vi "Flush if true.vi"(8 "error in":errorcluster, 10 "Bytes at port > X":bool, 11 "port in":refnum<visa-resource-name>) -> (0 "error out":errorcluster, 3 "port out":refnum<visa-resource-name>)   [LabVIEW 2013]
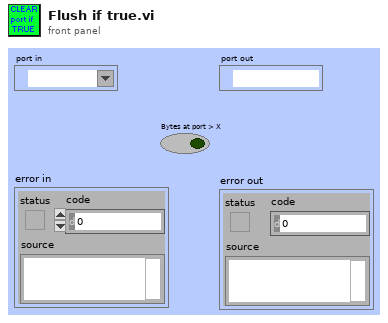
[diagram p1: front panel]
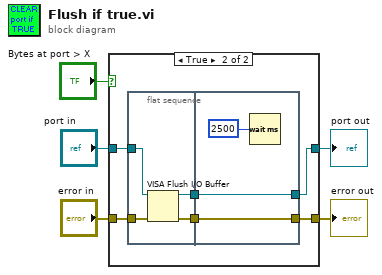
[diagram p0: block diagram]
diagram:
  n1 = case shown="True" "Bytes at port > X" {
    tunnel: [w7 w13] -> w1
    tunnel: "error in" -> [w7 w11]
    tunnel: "port in" -> [w6 w10]
    tunnel: [w6 w8] -> w5
    frame False {
    }
    frame True {
      n2 = flat-sequence {
        tunnel: [w17] -> w12
        tunnel: w11 -> [w16]
        tunnel: w10 -> [w15]
        tunnel: [w14] -> w9
        tunnel: [w19] -> w13
        tunnel: w12 -> [w19]
        tunnel: [w18] -> w8
        tunnel: w9 -> [w18]
        frame #0 {
          n3 = VISA Flush I/O Buffer(VISA resource name=w15, error in (no error)=w16) -> (VISA resource name out=w14:refnum<visa-resource-name>, error out=w17:errorcluster)  [unwired: 1 out]
        }
        frame #1 {
          n4 = Wait (ms)(milliseconds to wait=u32 2500) -> ()  [unwired: 1 out]
        }
      }
    }
  }
  "port out" <- w5
  "error out" <- w1
